vi "LimitFlagAction.vi"(4 "Axis limit flag":bool, 5 "Global limit flag active":dbl, 6 "Stop motors global":bool, 7 "Stop motor local":bool, 8 "Axis control signal":dbl) -> (0 "Slider control":dbl, 1 "PWM Brake":u32, 2 "PWM Direction":u32, 3 "PWM width":u32)   [LabVIEW 2009]
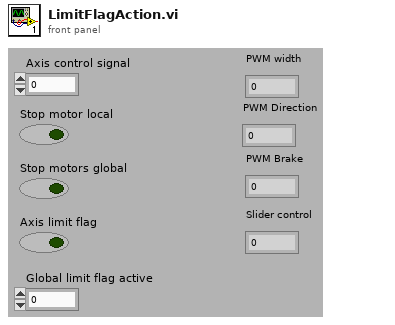
[diagram p1: front panel]
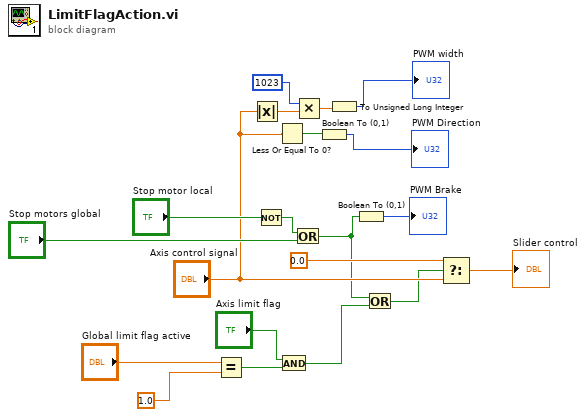
[diagram p0: block diagram]
diagram:
  n1 = Equal?(x="Global limit flag active", y=1.0) -> (x = y?=w18:bool)
  n2 = Absolute Value(x="Axis control signal") -> (abs(x)=w11:dbl)
  n3 = Not(x="Stop motor local") -> (.not. x?=w20:bool)
  n4 = Less Or Equal To 0?(x="Axis control signal") -> (x <= 0?=w8:bool)
  n5 = And(x="Axis limit flag", y=w18) -> (x .and. y?=w3:bool)
  n6 = Or(x=w20, y="Stop motors global") -> (x .or. y?=w2:bool)
  n7 = Multiply(x=1023, y=w11) -> (x*y=w9:dbl)
  n8 = Boolean To (0,1)(Boolean=w8) -> (0, 1=→"PWM Direction":i16)
  n9 = To Unsigned Long Integer(number=w9) -> (unsigned 32bit integer=→"PWM width":u32)
  n10 = Boolean To (0,1)(Boolean=w2) -> (0, 1=→"PWM Brake":i16)
  n11 = Or(x=w2, y=w3) -> (x .or. y?=w4:bool)
  n12 = Select(t=0.0, s=w4, f="Axis control signal") -> (s? t:f=→"Slider control":dbl)
